vi "Call Class Method.vi"(8 "error in (no error)":errorcluster) -> (0 "error out":errorcluster)   [LabVIEW 2020]
uses:
  b73fc05d-a0f2-49e8-8aed-f00845f7a653.vi
  a754d42d-cbdf-4b78-8a20-29fad82278de.vi
  G-Embedded-Python-Interpreter-Toolkit/Null Py Object Refnum.vi
  b73fc05d-a0f2-49e8-8aed-f00845f7a653.vi/96ddca92-7bbf-40e2-a1a5-d32f291eb6af.vi
  a754d42d-cbdf-4b78-8a20-29fad82278de.vi/6c7a13f1-33d3-431d-8188-904cac5422b3.vi
  G-Embedded-Python-Interpreter-Toolkit/Pointer Sized Ref to Python Object Reference.vi
  G-Embedded-Python-Interpreter-Toolkit/Generate Argument Type Info.vi
  G-Embedded-Python-Interpreter-Toolkit/Python Object Reference to Pointer Sized Ref.vi
  G-Embedded-Python-Interpreter-Toolkit/Variant to Type Info.vi
  G-Embedded-Python-Interpreter-Toolkit/Bad Type Error.vi
  G-Embedded-Python-Interpreter-Toolkit/Variant to Type Info.vi/8cdebbe9-3e59-4fbe-97b0-695fa0ebc24d.vi
  G-Embedded-Python-Interpreter-Toolkit/Merge Call Library Errors.vi
  <vilib>/Utility/Data Type/Get Type Information.vi
  <vilib>/Utility/error.llb/Error Cluster From Error Code.vi
  <vilib>/Utility/Data Type/Get Array Information.vi
  <vilib>/Utility/Data Type/Get Cluster Information.vi
  <vilib>/addons/_JKI Toolkits/Caraya/classes/Assert/Assert Not Error.vi
  <vilib>/addons/_JKI Toolkits/Caraya/classes/Assert/Assert Equal Value and Type_Variant.vi
  <vilib>/Comparison/Equal/Equal Functor/Equal Functor.lvclass
  G-Embedded-Python-Interpreter-Toolkit/G-Embedded-Python-Interpreter-Toolkit.lvlib
  <vilib>/addons/_JKI Toolkits/Caraya/classes/Assert/Assert.lvclass
  <vilib>/addons/_JKI Toolkits/Caraya/classes/Test/Test.lvclass
panel:
  out "Value":i32
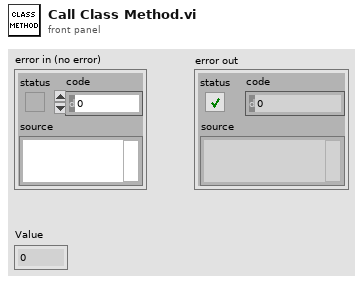
[diagram p1: front panel]
types:
  T1 = typedef "G-Embedded-Python-Interpreter-Toolkit.lvlib/Python Object Reference.ctl" = refnum<k1>
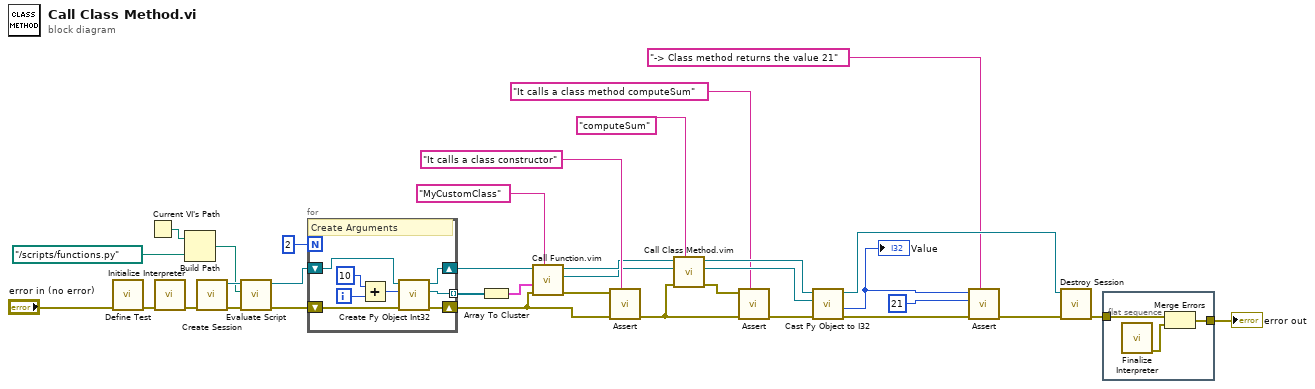
[diagram p0: block diagram]
diagram:
  n1 = call <vilib>:"Define Test.vi"("error in (no error)"="error in (no error)") -> ("error out"=w8:errorcluster)  [unwired: 10 in]
  n2 = Current VI's Path() -> (path=w32:path)
  n3 = call "Initialize Interpreter.vi"("error in (no error)"=w8) -> ("error out"=w34:errorcluster)  [unwired: 9 in, 1 out]
  n4 = Build Path(base path=w32, name or relative path=path "../scripts/functions.py" ("Path")) -> (appended path=w30:path)
  n5 = call "Create Session.vi"("error in (no error)"=w34) -> ("error out"=w29:errorcluster, "Session Handle"=w33:refnum<data-value>)  [unwired: 9 in]
  n6 = call "Evaluate Script.vi"("error in (no error)"=w29, "Script File Path"=w30, "Session Handle in"=w33) -> ("error out"=w26:errorcluster, "Session Handle out"=w27:refnum<data-value>)  [unwired: 7 in]
  n7 = for {
    N: 2 -> [_]
    shift-right: [w39] -> w25
    shift-left: w27 -> [w43]
    shift-right: [w40] -> w18
    shift-left: w26 -> [w42]
    tunnel: [w38] -> w6 mode=indexing
    i -> [w41]
    # "Create Arguments"
    n8 = Add(x=10, y=w41) -> (x+y=w37:i32)
    n9 = call "Create Py Object Int32.vi"("error in (no error)"=w42, "Value"=w37, "Session Handle in"=w43) -> ("error out"=w40:errorcluster, "Python Object Refnum"=w38:T1, "Session Handle out"=w39:refnum<data-value>)  [unwired: 6 in]
  }
  n10 = Array To Cluster(array=w6) -> (cluster=w5:cluster{"[0]":T1, "[1]":T1})
  n11 = call "Call Function.vim"("Function Name"="MyCustomClass", "error in (no error)"=w18, "Arguments in (Default - None)"=w5, "Data Value Reference in"=w25) -> ("error out"=w19:errorcluster, "Returned Python Object Refnum"=w3:T1, "Data Value Reference out"=w4:refnum<data-value>)  [unwired: 5 in]
  n12 = call-poly <vilib>:"Assert.vi"("Label"="It calls a class constructor", "error in (no error)"=w18, "Not Error?"=w19) -> ("error out"=w2:errorcluster)  [unwired: 8 in]
  n13 = call "Call Class Method.vim"("Function Name"="computeSum" ("Function/Method Name"), "error in (no error)"=w2, "Class Instance"=w3, "Data Value Reference in"=w4) -> ("error out"=w16:errorcluster, "Returned Python Object Refnum"=w21:T1, "Data Value Reference out"=w22:refnum<data-value>)  [unwired: 5 in]
  n14 = call-poly <vilib>:"Assert.vi"("Label"="It calls a class method computeSum", "error in (no error)"=w2, "Not Error?"=w16) -> ("error out"=w11:errorcluster)  [unwired: 8 in]
  n15 = call "Cast Py Object to I32.vi"("error in (no error)"=w11, "Python Object Refnum in"=w21, "Session Handle in"=w22) -> ("error out"=w10:errorcluster, "Value"=w14:i32, "Session Handle out"=w23:refnum<data-value>)  [unwired: 5 in, 1 out]
  "Value" <- w14
  n16 = call-poly <vilib>:"Assert.vi"("Label"="-> Class method returns the value 21", "error in (no error)"=w10, "Y"=21 ("Value"), "X"=w14) -> ("error out"=w12:errorcluster)  [unwired: 7 in]
  n17 = call "Destroy Session.vi"("error in (no error)"=w12, "Session Handle"=w23) -> ("error out"=w28:errorcluster)  [unwired: 9 in]
  n18 = flat-sequence {
    tunnel: w28 -> [w46]
    tunnel: [w44] -> w35
    frame #0 {
      n19 = call "Finalize Interpreter.vi"() -> ("error out"=w45:errorcluster)  [unwired: 11 in]
      n20 = Merge Errors(w46, w45) -> (w44:errorcluster)
    }
  }
  "error out" <- w35
